vi "Add All Child.vi"(8 "error in":errorcluster, 10 "Item in":refnum<class "Item.lvclass">, 11 "Parent Ref in":T1 format="%.0x") -> (0 "error out":errorcluster, 2 "Item out":refnum<class "Item.lvclass">, 3 "Parent Ref out":T1 format="%.0x")   [LabVIEW 2024, in "FPGA Addon System Explorer.lvlib"]
uses:
  FPGA Addon System Explorer.lvlib
  <vilib>/NI VeriStand/Custom Device API/Custom Device Item Ref.ctl
  Parser/Item/Item.lvclass
  Parser/Section/Section.lvclass
  Parser/Channel/Channel.lvclass
  <vilib>/NI VeriStand/Custom Device API/Custom Device API.lvlib
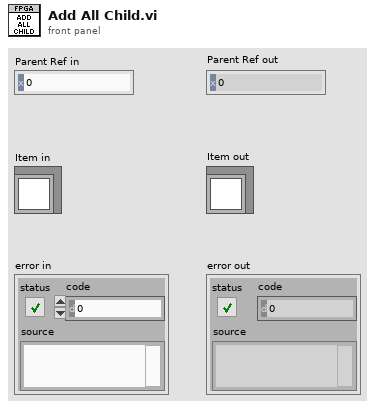
[diagram p1: front panel]
types:
  T1 = typedef "Custom Device API.lvlib/Custom Device Item Ref.ctl" = u64
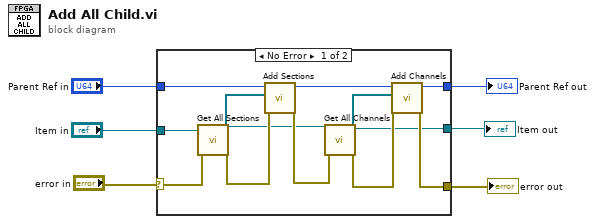
[diagram p0: block diagram]
diagram:
  n1 = case shown="No Error" "error in" {
    selector: "error in" -> [w15 w22]
    tunnel: [w16 w22] -> w6
    tunnel: "Item in" -> [w14 w20]
    tunnel: "Parent Ref in" -> [w13 w21]
    tunnel: [w9 w21] -> w2
    tunnel: [w8 w20] -> w1
    frame No Error {
      n2 = call "Get All Sections.vi"("error in"=w15, "Item in"=w14) -> ("error out"=w19:errorcluster, "Sections out"=w11:refnum<class "Section.lvclass">[], "Item out"=w12:refnum<class "Item.lvclass">)  [unwired: 7 in]
      n3 = call "Add Sections.vi"("error in"=w19, "Section in"=w11, "Node Ptr in"=w13) -> ("error out"=w18:errorcluster, "Node Ptr out"=w10:T1)  [unwired: 7 in]
      n4 = call "Get All Channels.vi"("error in"=w18, "Item in"=w12) -> ("error out"=w17:errorcluster, "Channels out"=w7:refnum<class "Channel.lvclass">[], "Item out"=w8:refnum<class "Item.lvclass">)  [unwired: 7 in]
      n5 = call "Add Channels.vi"("error in"=w17, "Channel in"=w7, "Node Ptr in"=w10) -> ("error out"=w16:errorcluster, "Node Ptr out"=w9:T1)  [unwired: 7 in]
    }
    frame Error {
    }
  }
  "error out" <- w6
  "Parent Ref out" <- w2
  "Item out" <- w1
